vi "min sample rate tester.vi"() -> ()   [LabVIEW 2013]
uses:
  LabVIEW/git_repos/Accelerator/Database2.0/Private/Unused/PSU updated.vi
panel:
  out "error out":errorcluster
  in  "min sample rate":dbl=1000000.0 format="%.2p"
  in  "stop":bool
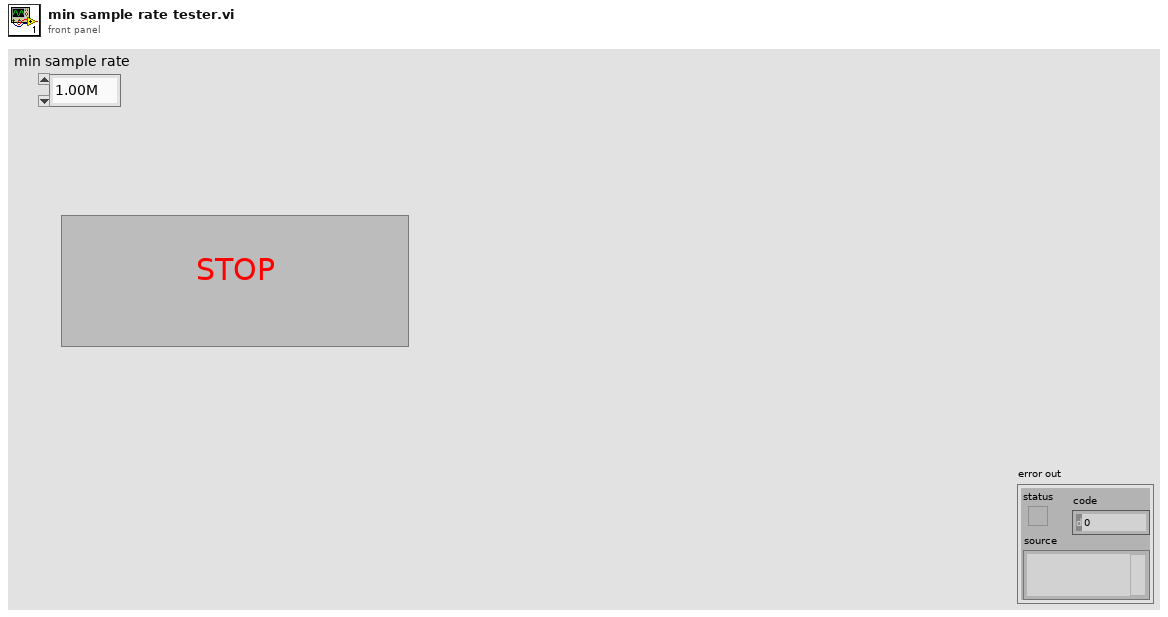
[diagram p1: front panel]
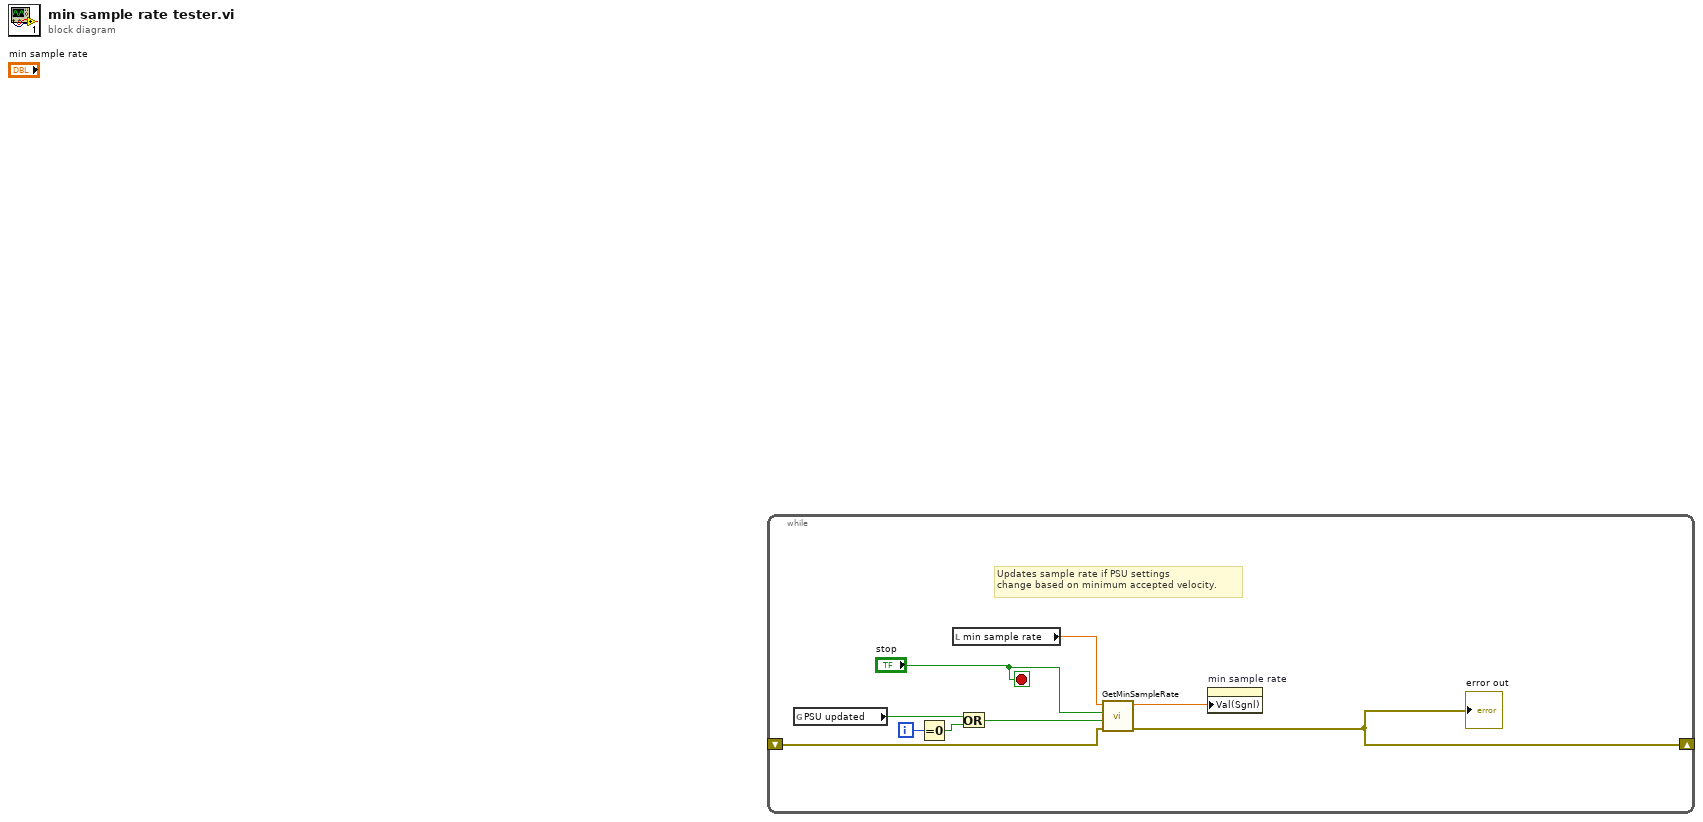
[diagram p0: block diagram]
diagram:
  n1 = while {
    shift-right: [w1] -> _
    shift-left: _ -> [w6]
    i -> [w9]
    stop <- "stop" stop-if-true
    # "Updates sample rate if PSU settings \nchange based on minimum accepted velocity."
    n2 = global read "PSU updated.vi" "PSU updated"() -> (w8:bool)
    n3 = Equal To 0?(x=w9) -> (x = 0?=w7:bool)
    n4 = local read "min sample rate"() -> (w4:dbl)
    n5 = Or(x=w8, y=w7) -> (x .or. y?=w5:bool)
    n6 = call "GetMinSampleRate.vi"("error in (no error)"=w6, "PSU Update"=w5, "stop"="stop", "min sample rate"=w4) -> ("error out"=w1:errorcluster, "min sample rate"=w3:dbl)  [unwired: 6 in]
    "error out" <- w1
    n7 = property on="min sample rate" class="DigNum (strict)"("Val(Sgnl)"=w3) -> ()  [unwired: 2 in, 2 out]
  }
